vi "Engine - Read Properties.vi"(8 "error in (no error)":errorcluster, 10 "DMM-Switch Configuration In":T1={"DMM Resource Name"="", "DMM Measurement"=enum."DC Volts", "DMM Resolution in Digits"=6.5, "DMM Range [EU]"=10.0, "DMM Temp - Value"={"DMM Temp - Transducer Type"=1, "DMM Temp - Thermocouple Type"=6, "DMM Temp - Fixed Reference Junction"=25.0, "DMM Temp - RTD Type"=enum."Pt3851", "DMM Temp - RTD Resistance"=100.0, "DMM Temp - Thermistor Type"=enum."44006", "DMM Temp - RTD A"=0.0039083, "DMM Temp - RTD B"=-5.775e-07, "DMM Temp - RTD C"=-4.183e-12, "DMM Temp - Thermistor A"=0.0010295, "DMM Temp - Thermistor B"=0.0002391, "DMM Temp - Thermistor C"=1.568e-07}, "Switch Resource Name"="", "Switch Topology"="2503/2-Wire 24x1 Mux", "Switch Scan List"="ab0->com0 & com0->ch0:2;", "Switch Trigger Source"=enum."TTL0", "Switch Scan Advanced Output"=enum."TTL1", "DMM Measurement Complete"=enum."TTL 0", "DMM Trigger Source"=enum."TTL 1", "# of Channels"=0, "Group CH Names - Configuration"="", "Group CH Names - Input Channels"="", "Group CH Names - Measurement Channels"="", "Group CH Names - Runtime Status"=""} {"DMM Temp - Value"."DMM Temp - Thermistor C" format="%#_13g"; "DMM Temp - Value"."DMM Temp - Thermistor B" format="%#_13g"; "DMM Temp - Value"."DMM Temp - Thermistor A" format="%#_13g"; "DMM Temp - Value"."DMM Temp - RTD Resistance" format="%.2f"; "DMM Temp - Value"."DMM Temp - Fixed Reference Junction" format="%.2f"; "DMM Temp - Value"."DMM Temp - Thermocouple Type" items=["B"=1, "E"=4, "J"=6, "K"=7, "N"=8, "R"=9, "S"=10, "T"=11]; "DMM Temp - Value"."DMM Temp - Transducer Type" items=["Thermocouple"=1, "Thermistor"=2, "2-Wire RTD"=3, "4-Wire RTD"=4]; "DMM Resolution in Digits" items=["3 1/2"=3.5, "4 1/2"=4.5, "5 1/2"=5.5, "6 1/2"=6.5, "7 1/2"=7.5]}, 11 "Specified Channel Ref List In":T14[](array[typedef]) format="%.0x") -> (0 "error out":errorcluster, 2 "DMM-Switch Configuration Out":T1={"DMM Resource Name"="", "DMM Measurement"=enum."DC Volts", "DMM Resolution in Digits"=0.0, "DMM Range [EU]"=0.0, "DMM Temp - Value"={"DMM Temp - Transducer Type"=1, "DMM Temp - Thermocouple Type"=6, "DMM Temp - Fixed Reference Junction"=25.0, "DMM Temp - RTD Type"=enum."Pt3851", "DMM Temp - RTD Resistance"=100.0, "DMM Temp - Thermistor Type"=enum."44006", "DMM Temp - RTD A"=0.0039083, "DMM Temp - RTD B"=-5.775e-07, "DMM Temp - RTD C"=-4.183e-12, "DMM Temp - Thermistor A"=0.0010295, "DMM Temp - Thermistor B"=0.0002391, "DMM Temp - Thermistor C"=1.568e-07}, "Switch Resource Name"="", "Switch Topology"="", "Switch Scan List"="", "Switch Trigger Source"=enum."Immediate", "Switch Scan Advanced Output"=enum."None", "DMM Measurement Complete"=enum."None", "DMM Trigger Source"=enum."Immediate", "# of Channels"=0, "Group CH Names - Configuration"="", "Group CH Names - Input Channels"="", "Group CH Names - Measurement Channels"="", "Group CH Names - Runtime Status"=""} {"DMM Temp - Value"."DMM Temp - Thermistor C" format="%#_13g"; "DMM Temp - Value"."DMM Temp - Thermistor B" format="%#_13g"; "DMM Temp - Value"."DMM Temp - Thermistor A" format="%#_13g"; "DMM Temp - Value"."DMM Temp - RTD Resistance" format="%.2f"; "DMM Temp - Value"."DMM Temp - Fixed Reference Junction" format="%.2f"; "DMM Temp - Value"."DMM Temp - Thermocouple Type" items=["B"=1, "E"=4, "J"=6, "K"=7, "N"=8, "R"=9, "S"=10, "T"=11]; "DMM Temp - Value"."DMM Temp - Transducer Type" items=["Thermocouple"=1, "Thermistor"=2, "2-Wire RTD"=3, "4-Wire RTD"=4]; "DMM Resolution in Digits" items=["3 1/2"=3.5, "4 1/2"=4.5, "5 1/2"=5.5, "6 1/2"=6.5, "7 1/2"=7.5]}, 3 "Specified Channel Ref List Out":T14[](array[typedef]) format="%.0x")   [LabVIEW 2016, in "DMM-SWITCH-ScanList Engine.lvlib"]
doc: "Reads all properties from Input Configuration Channels (DMM, Switch, and Triggering) and writes them into the DMM-Switch Configuration Cluster"
uses:
  DMM-SWITCH-ScanList Engine.lvlib
  TypeDefs/DMM-Switch Configuration.ctl
  <instrlib>/niDMM/nidmm.llb/niDMM Function.ctl
  <instrlib>/niDMM/nidmm.llb/niDMM Resolution in Digits.ctl
  System Explorer/Pages/Configuration Controls/DMM Temp.ctl
  <instrlib>/niDMM/nidmm.llb/niDMM Transducer Type.ctl
  <instrlib>/niDMM/nidmm.llb/niDMM Thermocouple Type.ctl
  <instrlib>/niDMM/nidmm.llb/niDMM RTD Type.ctl
  <instrlib>/niDMM/nidmm.llb/niDMM Thermistor Type.ctl
  <instrlib>/niSwitch/niSwitch.llb/niSwitch Topologies.ctl
  <instrlib>/niSwitch/niSwitch.llb/niSwitch Trigger Input.ctl
  <instrlib>/niSwitch/niSwitch.llb/niSwitch Scan Advanced Output.ctl
  <instrlib>/niDMM/nidmm.llb/niDMM Measurement Complete.ctl
  <instrlib>/niDMM/nidmm.llb/niDMM Trigger.ctl
  <vilib>/NI Veristand/Custom Device API/Custom Device Item Ref.ctl
  Shared/Constants.vi
  <vilib>/NI Veristand/Custom Device API/Get Item Property (String).vi
  <vilib>/NI Veristand/Custom Device API/Get Item Property (String Array).vi
  <vilib>/NI Veristand/Custom Device API/Get Item Property (U16).vi
  <vilib>/NI Veristand/Custom Device API/Get Item Property (Double).vi
  <vilib>/NI Veristand/Custom Device API/Get Item Property (Variant).vi
  <vilib>/NI Veristand/Custom Device API/Custom Device API.lvlib
  Shared/DMM-SWITCH-ScanList Shared.lvlib
  System Explorer/DMM-SWITCH-ScanList System Explorer.lvlib
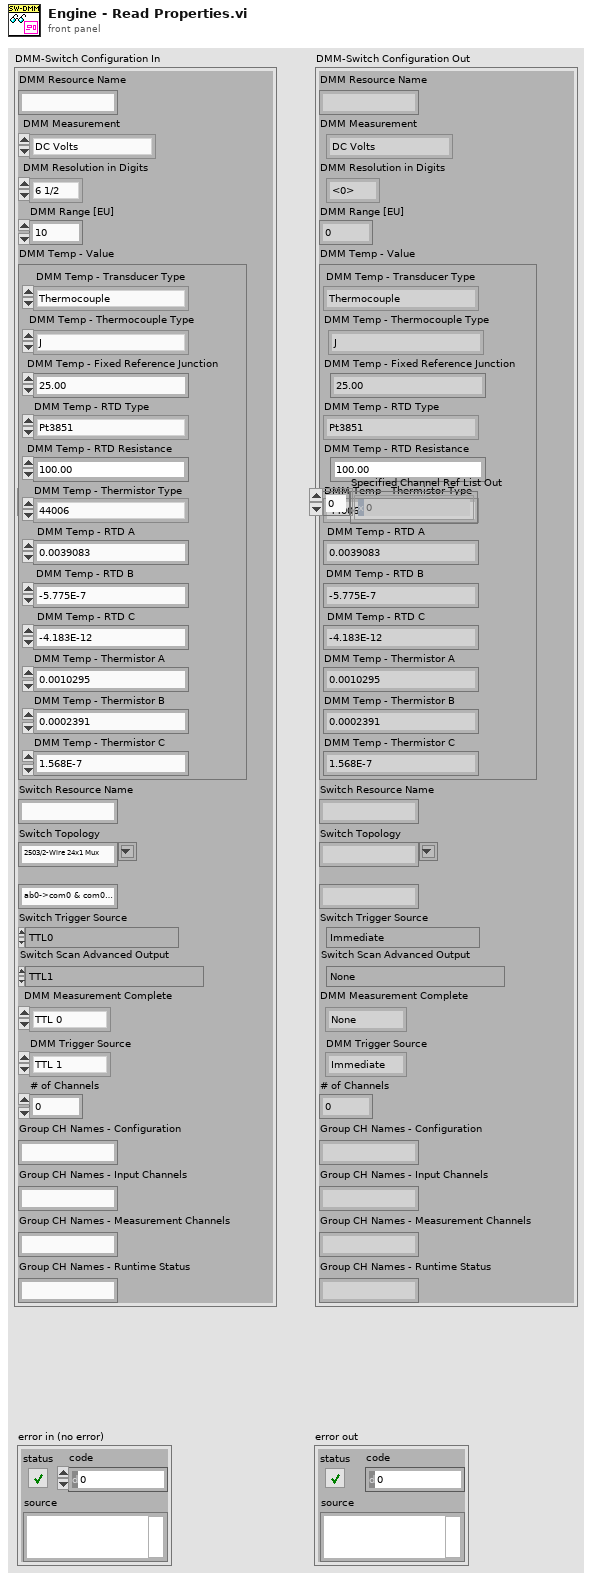
[diagram p1: front panel]
types:
  T1 = typedef "DMM-SWITCH-ScanList Engine.lvlib/DMM-Switch Configuration.ctl" = cluster{"DMM Resource Name":string, "DMM Measurement":T2, "DMM Resolution in Digits":T3, "DMM Range [EU]":dbl, "DMM Temp - Value":T4, "Switch Resource Name":string, "Switch Topology":T9, "Switch Scan List":string, "Switch Trigger Source":T10, "Switch Scan Advanced Output":T11, "DMM Measurement Complete":T12, "DMM Trigger Source":T13, "# of Channels":u32, "Group CH Names - Configuration":string, "Group CH Names - Input Channels":string, "Group CH Names - Measurement Channels":string, "Group CH Names - Runtime Status":string}
  T2 = typedef "niDMM Function.ctl" = enum16{"DC Volts", "AC Volts", "DC Current", "AC Current", "2-wire Resistance", "4-wire Resistance", "Diode", "Frequency", "Period", "AC Volts DC Coupled", "Capacitance", "Inductance", "Temperature"}
  T3 = typedef "niDMM Resolution in Digits.ctl" = dbl
  T4 = typedef "DMM-SWITCH-ScanList System Explorer.lvlib/DMM Temp.ctl" = cluster{"DMM Temp - Transducer Type":T5, "DMM Temp - Thermocouple Type":T6, "DMM Temp - Fixed Reference Junction":dbl, "DMM Temp - RTD Type":T7, "DMM Temp - RTD Resistance":dbl, "DMM Temp - Thermistor Type":T8, "DMM Temp - RTD A":dbl, "DMM Temp - RTD B":dbl, "DMM Temp - RTD C":dbl, "DMM Temp - Thermistor A":dbl, "DMM Temp - Thermistor B":dbl, "DMM Temp - Thermistor C":dbl}
  T5 = typedef "niDMM Transducer Type.ctl" = i32
  T6 = typedef "niDMM Thermocouple Type.ctl" = i32
  T7 = typedef "niDMM RTD Type.ctl" = enum16{"Custom", "Pt3750", "Pt3851", "Pt3911", "Pt3916", "Pt3920", "Pt3928"}
  T8 = typedef "niDMM Thermistor Type.ctl" = enum16{"Custom", "44004", "44006", "44007"}
  T9 = typedef "niSwitch Topologies.ctl" = string
  T10 = typedef "niSwitch Trigger Input.ctl" = enum16{"Immediate", "External", "TTL0", "TTL1", "TTL2", "TTL3", "TTL4", "TTL5", "TTL6", "TTL7", "ECL0", "ECL1", "PXI Star", "Software Trigger Function", "Rear Connector", "Front Connector", "Rear Connector of Module 1", "Rear Connector of Module 2", "Rear Connector of Module 3", "Rear Connector of Module 4", "Rear Connector of Module 5", "Rear Connector of Module 6", "Rear Connector of Module 7", "Rear Connector of Module 8", "Rear Connector of Module 9", "Rear Connector of Module 10", "Rear Connector of Module 11", "Rear Connector of Module 12", "Front Connector of Module 1", "Front Connector of Module 2", "Front Connector of Module 3", "Front Connector of Module 4", "Front Connector of Module 5", "Front Connector of Module 6", "Front Connector of Module 7", "Front Connector of Module 8", "Front Connector of Module 9", "Front Connector of Module 10", "Front Connector of Module 11", "Front Connector of Module 12"}
  T11 = typedef "niSwitch Scan Advanced Output.ctl" = enum16{"None", "External", "TTL0", "TTL1", "TTL2", "TTL3", "TTL4", "TTL5", "TTL6", "TTL7", "ECL0", "ECL1", "PXI Star", "Rear Connector", "Front Connector", "Rear Connector Module 1", "Rear Connector Module 2", "Rear Connector Module 3", "Rear Connector Module 4", "Rear Connector Module 5", "Rear Connector Module 6", "Rear Connector Module 7", "Rear Connector Module 8", "Rear Connector Module 9", "Rear Connector Module 10", "Rear Connector Module 11", "Rear Connector Module 12", "Front Connector Module 1", "Front Connector Module 2", "Front Connector Module 3", "Front Connector Module 4", "Front Connector Module 5", "Front Connector Module 6", "Front Connector Module 7", "Front Connector Module 8", "Front Connector Module 9", "Front Connector Module 10", "Front Connector Module 11", "Front Connector Module 12"}
  T12 = typedef "niDMM Measurement Complete.ctl" = enum16{"None", "External", "TTL 0", "TTL 1", "TTL 2", "TTL 3", "TTL 4", "TTL 5", "TTL 6", "TTL 7", "LBR Trig 0"}
  T13 = typedef "niDMM Trigger.ctl" = enum16{"Immediate", "External", "TTL 0", "TTL 1", "TTL 2", "TTL 3", "TTL 4", "TTL 5", "TTL 6", "Software", "TTL 7", "PXI Star", "LBR Trig 1", "Aux Trig 1"}
  T14 = typedef "Custom Device API.lvlib/Custom Device Item Ref.ctl" = u64
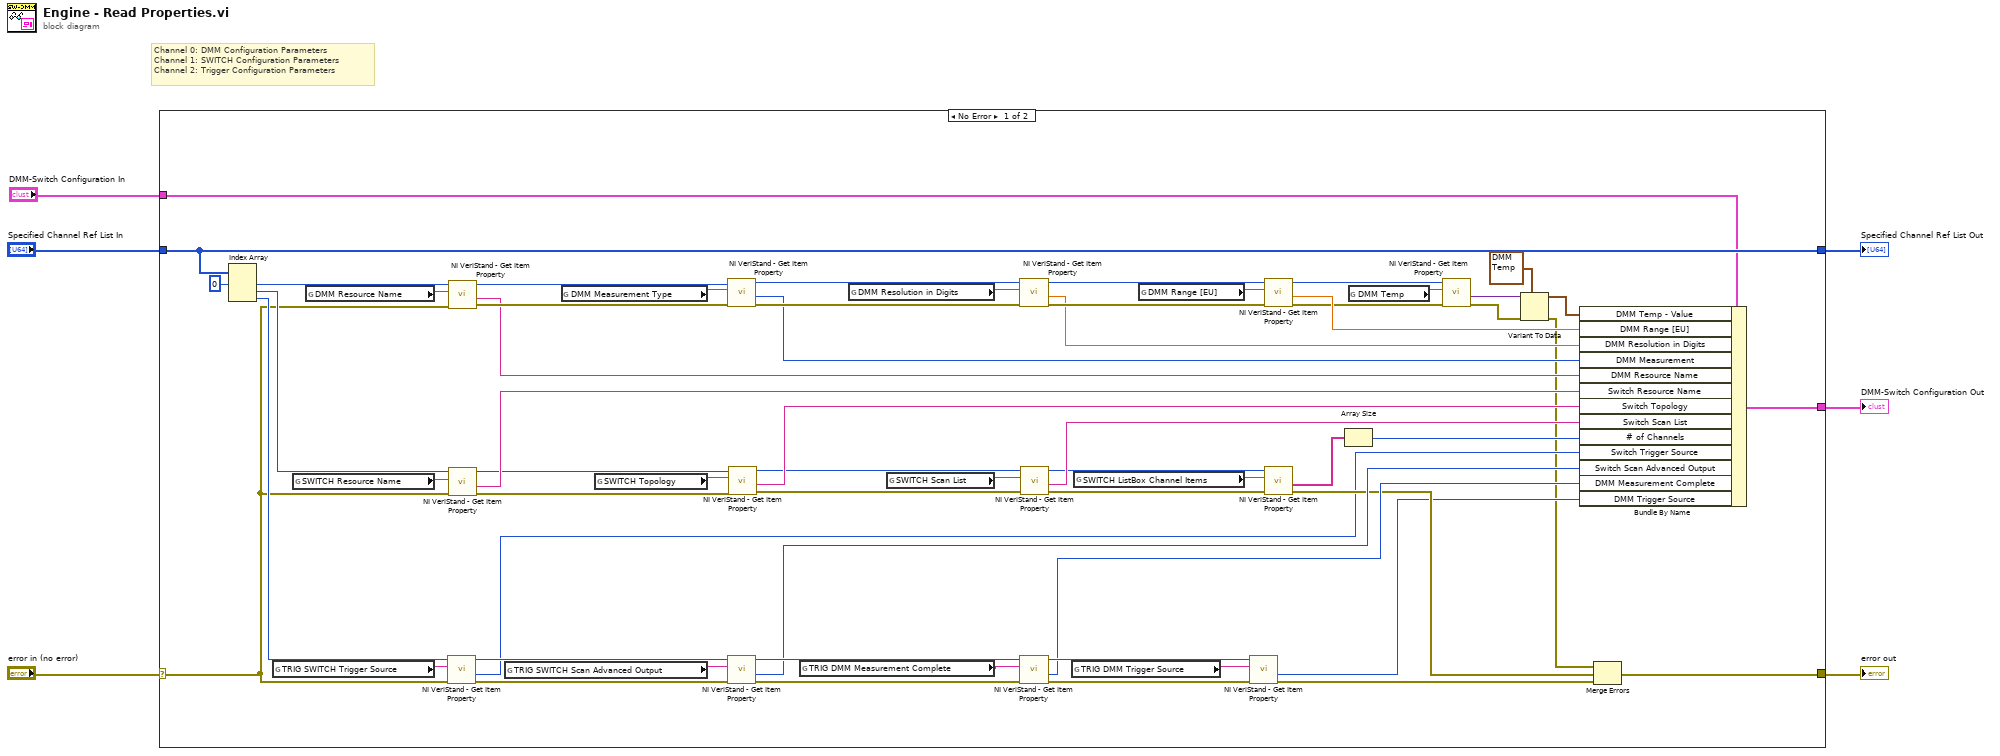
[diagram p0: block diagram]
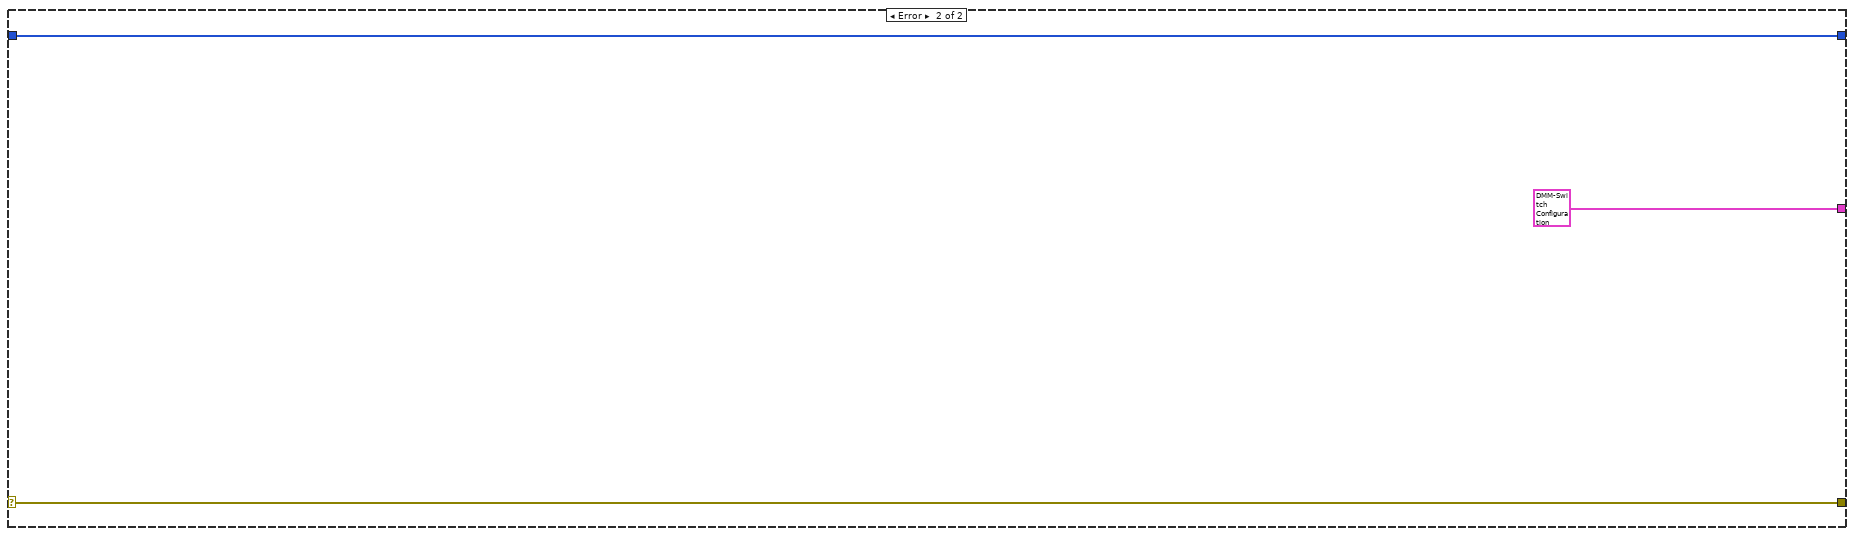
[diagram p2: hidden frame]
diagram:
  # "Channel 0: DMM Configuration Parameters\nChannel 1: SWITCH Configuration Parameters\nChannel 2: Trigger Configuration Parameters"
  n1 = case shown="No Error" "error in (no error)" {
    selector: "error in (no error)" -> [w41 w71]
    tunnel: [w67 w71] -> w6
    tunnel: [w66 T1 {"DMM Resource Name"="", "DMM Measurement"=enum."DC Volts", "DMM Resolution in Digits"=6.5, "DMM Range [EU]"=10.0, "DMM Temp - Value"={"DMM Temp - Transducer Type"=1, "DMM Temp - Thermocouple Type"=6, "DMM Temp - Fixed Reference Junction"=25.0, "DMM Temp - RTD Type"=enum."Pt3851", "DMM Temp - RTD Resistance"=100.0, "DMM Temp - Thermistor Type"=enum."44006", "DMM Temp - RTD A"=0.0039083, "DMM Temp - RTD B"=-5.775e-07, "DMM Temp - RTD C"=-4.183e-12, "DMM Temp - Thermistor A"=0.0010295, "DMM Temp - Thermistor B"=0.0002391, "DMM Temp - Thermistor C"=1.568e-07}, "Switch Resource Name"="", "Switch Topology"="2503/2-Wire 24x1 Mux", "Switch Scan List"="ab0->com0 & com0->ch0:2;", "Switch Trigger Source"=enum."TTL0", "Switch Scan Advanced Output"=enum."TTL1", "DMM Measurement Complete"=enum."TTL 0", "DMM Trigger Source"=enum."TTL 1", "# of Channels"=0, "Group CH Names - Configuration"="", "Group CH Names - Input Channels"="", "Group CH Names - Measurement Channels"="", "Group CH Names - Runtime Status"=""} ("DMM-Switch Configuration")] -> w5
    tunnel: "Specified Channel Ref List In" -> [w40 w70]
    tunnel: [w40 w70] -> w2
    tunnel: "DMM-Switch Configuration In" -> [w16 _]
    frame No Error {
      n2 = Index Array(array=w40, index #1=0 ("index")) -> (element #1=w49:T14, element #2=w57:T14, element #3=w58:T14)  [unwired: 2 in]
      n3 = global read "Constants.vi" "TRIG SWITCH Trigger Source"() -> (w30:string)
      n4 = global read "Constants.vi" "SWITCH Resource Name"() -> (w31:string)
      n5 = global read "Constants.vi" "DMM Resource Name"() -> (w32:string)
      n6 = call-poly <vilib>:"NI VeriStand - Get Item Property.vi"("error in (no error)"=w41, "Property Name"=w30, "Item Ref in"=w58) -> ("error out"=w55:errorcluster, "Value"=w36:u16, "Item Ref out"=w63:T14)  [unwired: 5 in, 1 out]
      n7 = call-poly <vilib>:"NI VeriStand - Get Item Property.vi"("error in (no error)"=w41, "Property Name"=w32, "Item Ref in"=w49) -> ("error out"=w48:errorcluster, "Value"=w18:string, "Item Ref out"=w47:T14)  [unwired: 5 in, 1 out]
      n8 = call-poly <vilib>:"NI VeriStand - Get Item Property.vi"("error in (no error)"=w41, "Property Name"=w31, "Item Ref in"=w57) -> ("error out"=w53:errorcluster, "Value"=w59:string, "Item Ref out"=w52:T14)  [unwired: 5 in, 1 out]
      n9 = global read "Constants.vi" "TRIG SWITCH Scan Advanced Output"() -> (w27:string)
      n10 = global read "Constants.vi" "DMM Measurement Type"() -> (w29:string)
      n11 = global read "Constants.vi" "SWITCH Topology"() -> (w28:string)
      n12 = call-poly <vilib>:"NI VeriStand - Get Item Property.vi"("error in (no error)"=w48, "Property Name"=w29, "Item Ref in"=w47) -> ("error out"=w45:errorcluster, "Value"=w19:u16, "Item Ref out"=w46:T14)  [unwired: 5 in, 1 out]
      n13 = call-poly <vilib>:"NI VeriStand - Get Item Property.vi"("error in (no error)"=w55, "Property Name"=w27, "Item Ref in"=w63) -> ("error out"=w56:errorcluster, "Value"=w61:u16, "Item Ref out"=w64:T14)  [unwired: 5 in, 1 out]
      n14 = call-poly <vilib>:"NI VeriStand - Get Item Property.vi"("error in (no error)"=w53, "Property Name"=w28, "Item Ref in"=w52) -> ("error out"=w50:errorcluster, "Value"=w68:string, "Item Ref out"=w51:T14)  [unwired: 5 in, 1 out]
      n15 = global read "Constants.vi" "TRIG DMM Measurement Complete"() -> (w26:string)
      n16 = global read "Constants.vi" "DMM Resolution in Digits"() -> (w24:string)
      n17 = global read "Constants.vi" "SWITCH Scan List"() -> (w25:string)
      n18 = call-poly <vilib>:"NI VeriStand - Get Item Property.vi"("error in (no error)"=w45, "Property Name"=w24, "Item Ref in"=w46) -> ("error out"=w43:errorcluster, "Value"=w20:dbl, "Item Ref out"=w44:T14)  [unwired: 5 in, 1 out]
      n19 = call-poly <vilib>:"NI VeriStand - Get Item Property.vi"("error in (no error)"=w56, "Property Name"=w26, "Item Ref in"=w64) -> ("error out"=w54:errorcluster, "Value"=w62:u16, "Item Ref out"=w65:T14)  [unwired: 5 in, 1 out]
      n20 = call-poly <vilib>:"NI VeriStand - Get Item Property.vi"("error in (no error)"=w50, "Property Name"=w25, "Item Ref in"=w51) -> ("error out"=w39:errorcluster, "Value"=w60:string, "Item Ref out"=w37:T14)  [unwired: 5 in, 1 out]
      n21 = global read "Constants.vi" "TRIG DMM Trigger Source"() -> (w17:string)
      n22 = global read "Constants.vi" "SWITCH ListBox Channel Items"() -> (w22:string)
      n23 = global read "Constants.vi" "DMM Range [EU]"() -> (w23:string)
      n24 = call-poly <vilib>:"NI VeriStand - Get Item Property.vi"("error in (no error)"=w54, "Property Name"=w17, "Item Ref in"=w65) -> ("error out"=w15:errorcluster, "Value"=w33:u16)  [unwired: 5 in, 2 out]
      n25 = call-poly <vilib>:"NI VeriStand - Get Item Property.vi"("error in (no error)"=w43, "Property Name"=w23, "Item Ref in"=w44) -> ("error out"=w12:errorcluster, "Value"=w21:dbl, "Item Ref out"=w14:T14)  [unwired: 5 in, 1 out]
      n26 = call-poly <vilib>:"NI VeriStand - Get Item Property.vi"("error in (no error)"=w39, "Property Name"=w22, "Item Ref in"=w37) -> ("error out"=w38:errorcluster, "Value"=w35:string[])  [unwired: 5 in, 2 out]
      n27 = Array Size(array=w35) -> (size(s)=w34:i32)
      n28 = global read "Constants.vi" "DMM Temp"() -> (w13:string)
      n29 = call-poly <vilib>:"NI VeriStand - Get Item Property.vi"("error in (no error)"=w12, "Property Name"=w13, "Item Ref in"=w14) -> ("error out"=w8:errorcluster, "Value"=w10:variant)  [unwired: 5 in, 2 out]
      n30 = Variant To Data(error in=w8, type=T4 {"DMM Temp - Transducer Type"=1, "DMM Temp - Thermocouple Type"=6, "DMM Temp - Fixed Reference Junction"=25.0, "DMM Temp - RTD Type"=enum."Pt3851", "DMM Temp - RTD Resistance"=100.0, "DMM Temp - Thermistor Type"=enum."44006", "DMM Temp - RTD A"=0.0039083, "DMM Temp - RTD B"=-5.775e-07, "DMM Temp - RTD C"=-4.183e-12, "DMM Temp - Thermistor A"=0.0010295, "DMM Temp - Thermistor B"=0.0002391, "DMM Temp - Thermistor C"=1.568e-07} ("DMM Temp - Value"), Variant=w10) -> (data=w9:T4, error out=w7:errorcluster)
      n31 = Bundle By Name(cluster=w16, "DMM Temp - Value"=w9, "DMM Range [EU]"=w21, "DMM Resolution in Digits"=w20, "DMM Measurement"=w19, "DMM Resource Name"=w18, "Switch Resource Name"=w59, "Switch Topology"=w68, "Switch Scan List"=w60, "# of Channels"=w34, "Switch Trigger Source"=w36, "Switch Scan Advanced Output"=w61, "DMM Measurement Complete"=w62, "DMM Trigger Source"=w33) -> (w66:T1)
      n32 = Merge Errors(w7, w38, w15) -> (w67:errorcluster)
    }
    frame Error {
    }
  }
  "error out" <- w6
  "DMM-Switch Configuration Out" <- w5
  "Specified Channel Ref List Out" <- w2
